vi "RAMP_single_scan_FPGA.vi"(4 "error in":errorcluster, 5 "Ramp":dbl[](array[numeric]), 6 "queue piezo":refnum<queue>, 7 "queue DAQ":refnum<queue>) -> (0 "error out":errorcluster)   [LabVIEW 2015]
uses:
  CONTROLS/Q_MCL_piezo_element.ctl
  CONTROLS/Q_DAQ_element.ctl
  GLOBAL/Global_ABORT.vi
  GLOBAL/Global_MAIN.vi
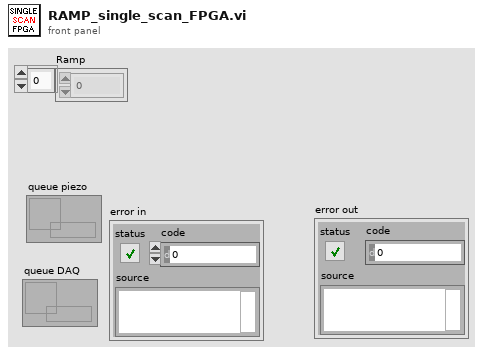
[diagram p1: front panel]
types:
  T1 = typedef "Q_DAQ_element.ctl" = cluster{"variant":variant, "Instruction":enum16{"DAQ_idle", "DAQ_initialize", "DAQ_error", "DAQ_security_stop", "DAQ_init_single_scan", "DAQ_single_scan", "DAQ_init_merFISH", "DAQ_scan_merFISH", "DAQ_photobleaching_merFISH", "DAQ_close_merFISH", "DAQ_stop"}}
  T2 = typedef "Q_MCL_piezo_element.ctl" = cluster{"variant":variant, "Instruction":enum16{"Piezo_idle", "Piezo_initialize", "Piezo_error", "Piezo_security_stop", "Piezo_read_z", "Piezo_move_z", "Piezo_keyboard_move", "Piezo_close_autofocus_calibration_ramp", "Piezo_change_init_state", "Piezo_init_autofocus", "Piezo_init_autofocus_merFISH_TL", "Piezo_autofocus", "Piezo_autofocus_merFISH_TL", "Piezo_stop_autofocus", "Piezo_stop_autofocus_merFISH_TL", "Piezo_autofocus_lost", "Piezo_resume_autofocus_merFISH_TL", "Piezo_check_z_position_merFISH_TL", "Piezo_init_ramp", "Piezo_move_z_ramp", "Piezo_close_ramp", "Piezo_close_merFISH", "Piezo_stop"}}
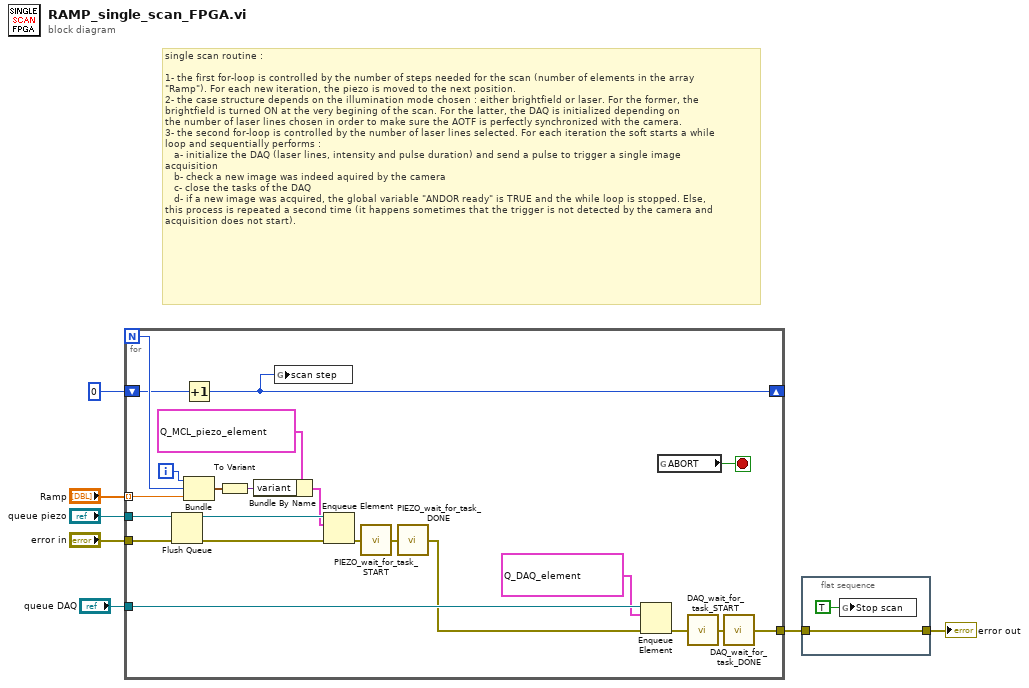
[diagram p0: block diagram]
diagram:
  # "single scan routine :\n\n1- the first for-loop is controlled by the number of steps needed for the scan (number of elements in the array\n\"Ramp\"). For each new iteration, the piezo is moved to the next position.\n2- the case structure depends on the illumination mode chosen : either brightfield or laser. For the former, the\nbrightfield is turned ON at the very begining of the scan. For the latter, the DAQ is initialized depending on\nthe number of laser lines chosen in order to make sure the AOTF is perfectly synchronized with the camera.\n3- the second for-loop is controlled by the number of laser lines selected. For each iteration the soft starts a while\nloop and sequentially performs :\n   a- initialize the DAQ (laser lines, intensity and pulse duration) and send a pulse to trigger a single image\nacquisition\n   b- check a new image was indeed aquired by the camera\n   c- close the tasks of the DAQ\n   d- if a new image was acquired, the global variable \"ANDOR ready\" is TRUE and the while loop is stopped. Else, \nthis process is repeated a second time (it happens sometimes that the trigger is not detected by the camera and\nacquisition does not start)."
  n1 = for {
    N -> [w17]
    tunnel: "Ramp" -> [w19] mode=indexing
    tunnel: "queue piezo" -> [w29]
    shift-right: [w15] -> _
    shift-left: 0 -> [w16]
    tunnel: "error in" -> [w9]
    tunnel: "queue DAQ" -> [w14]
    tunnel: [w8] -> w1
    i -> [w18]
    stop <- w21 stop-if-true
    n2 = Flush Queue(queue=w29, error in (no error)=w9) -> (queue out=w26:refnum<queue>, error out=w25:errorcluster)  [unwired: 1 out]
    n3 = Increment(x=w16) -> (x+1=w15:i32)
    n4 = Bundle(w18, w17, w19) -> (w20:cluster{i32, i32, dbl})  [unwired: 1 in]
    n5 = To Variant(anything=w20) -> (Variant=w27:variant)
    n6 = Bundle By Name(cluster=T2 {"variant"=variant, "Instruction"=enum."Piezo_move_z_ramp"} ("Q_MCL_Piezo"), "variant"=w27) -> (w24:T2)
    n7 = global write "Global_MAIN.vi" "scan step"(w15) -> ()
    n8 = Enqueue Element(queue=w26, element=w24, error in (no error)=w25) -> (error out=w23:errorcluster)  [unwired: 1 in, 2 out]
    n9 = call "PIEZO_wait_for_task_START.vi"("error in"=w23) -> ("error out"=w22:errorcluster)
    n10 = call "PIEZO_wait_for_task_DONE.vi"("error in"=w22) -> ("error out"=w13:errorcluster)
    n11 = Enqueue Element(queue=w14, element=T1 {"variant"=variant, "Instruction"=enum."DAQ_single_scan"}, error in (no error)=w13) -> (error out=w12:errorcluster)  [unwired: 1 in, 2 out]
    n12 = global read "Global_ABORT.vi" "ABORT"() -> (w21:bool)
    n13 = call "DAQ_wait_for_task_START.vi"("error in"=w12) -> ("error out"=w11:errorcluster)
    n14 = call "DAQ_wait_for_task_DONE.vi"("error in"=w11) -> ("error out"=w8:errorcluster)
  }
  n15 = flat-sequence {
    tunnel: [w30] -> w2
    tunnel: w1 -> [w30]
    frame #0 {
      n16 = global write "Global_MAIN.vi" "Stop scan"(TRUE ("Stop scan")) -> ()
    }
  }
  "error out" <- w2
